vi "Write Port.vi"(8 "error in (no error)":errorcluster, 10 "Data":u8, 11 "Handle":u32) -> (0 "error out":errorcluster, 3 "Status":i32)   [LabVIEW 2016, in "Drivers.lvlib" / "C8855-01.lvlib"]
doc: "Write 2-bit data into the general-purpose output port on this unit. Valid only for lower 2 bits of data. Set 0 in the upper 6 bits. Use this output signal for controlling external equipment.\n\n\n\nBOOL C8855API __stdcall C8855WritePort( HANDLE hC8855,\n BYTE Data );"
uses:
  C8855-01.lvlib
  C8855-01api.dll
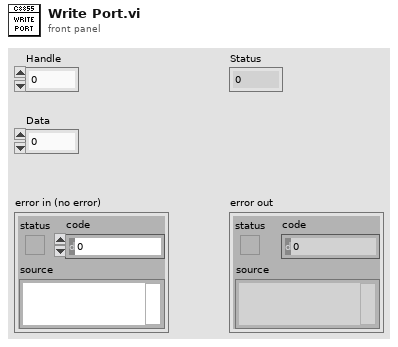
[diagram p1: front panel]
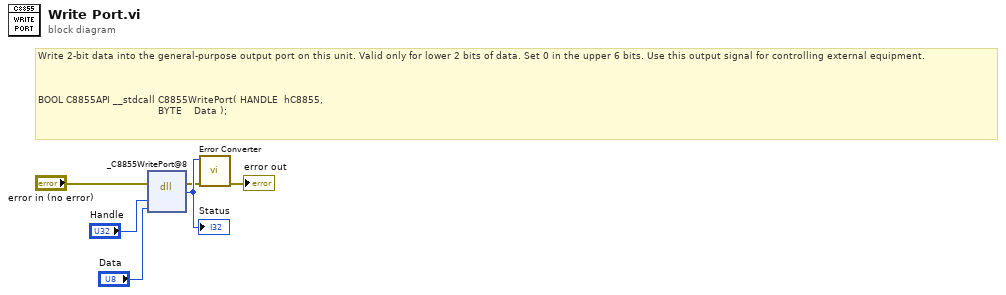
[diagram p0: block diagram]
diagram:
  # "Write 2-bit data into the general-purpose output port on this unit. Valid only for lower 2 bits of data. Set 0 in the upper 6 bits. Use this output signal for controlling external equipment.\n\n\n\nBOOL C8855API __stdcall C8855WritePort( HANDLE  hC8855,\n                                        BYTE    Data );"
  n1 = dll-call lib="Z:/TraceGrabber/Drivers/C8855-01/C8855-01api.dll" fn="_C8855WritePort@8"(error in="error in (no error)", "Handle"="Handle", "Data"="Data") -> (error out=w2:errorcluster, "return type"=w6:i32)  [unwired: 4 in, 1 out]
  "Status" <- w6
  n2 = call "Error Converter.vi"("error in (no error)"=w2, "error code"=w6) -> ("error out"=→"error out":errorcluster)  [unwired: 9 in]
